vi "Write Connect Parameter.vi"(8 "error in (no error)":errorcluster, 10 "Connect Parameter":T2={"IO Card Type"=enum."None", "IOType"=enum."Output", "CardNumber"=0, "ConnectAct"=FALSE, "IP"=""}, 11 "IOCard in":refnum<class "IOCard.lvclass">) -> (0 "error out":errorcluster, 3 "IOCard out":refnum<class "IOCard.lvclass">)   [LabVIEW 2019, in "IOCard.lvclass"]
uses:
  IOCard.lvclass
  IO_VI/IOCtrl/Ctrl/IO Card_Type.ctl
  IOCard.lvclass/IOCard.ctl
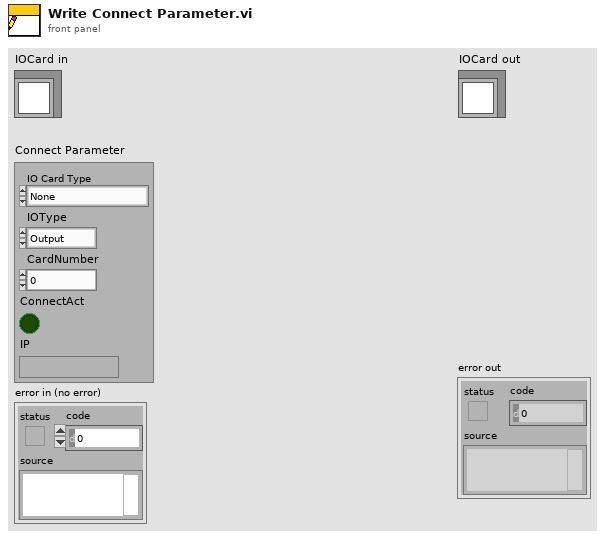
[diagram p1: front panel]
types:
  T1 = typedef "IO Card_Type.ctl" = enum16{"None", "Unidaq32", "6480", "2410C-64", "Zan", "DMC1000B", "16InOut", "Robot", "DMC3600"}
  T2 = cluster{"IO Card Type":T1, "IOType":enum16{"Input", "Output"}, "CardNumber":i32, "ConnectAct":bool, "IP":string}
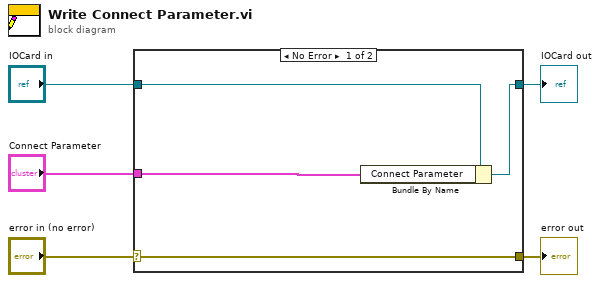
[diagram p0: block diagram]
diagram:
  n1 = case shown="No Error" "error in (no error)" {
    selector: "error in (no error)" -> [w9 w10]
    tunnel: [w9 w10] -> w4
    tunnel: [w7 w11] -> w2
    tunnel: "IOCard in" -> [w8 w11]
    tunnel: "Connect Parameter" -> [w6 _]
    frame No Error {
      n2 = Bundle By Name(cluster=w8, "Connect Parameter"=w6) -> (w7:refnum<class "IOCard.lvclass">)
    }
    frame Error {
    }
  }
  "error out" <- w4
  "IOCard out" <- w2
